vi "initializeArrayElement.vi"(8 "error in (no error)":errorcluster, 9 "arraySize":u16, 10 "arrayRef":refnum<vi>, 11 "Boolean in":refnum<class "Boolean.lvclass">) -> (0 "error out":errorcluster, 3 "Boolean out":refnum<class "Boolean.lvclass">)   [LabVIEW 2016, in "Boolean.lvclass"]
uses:
  Boolean.lvclass
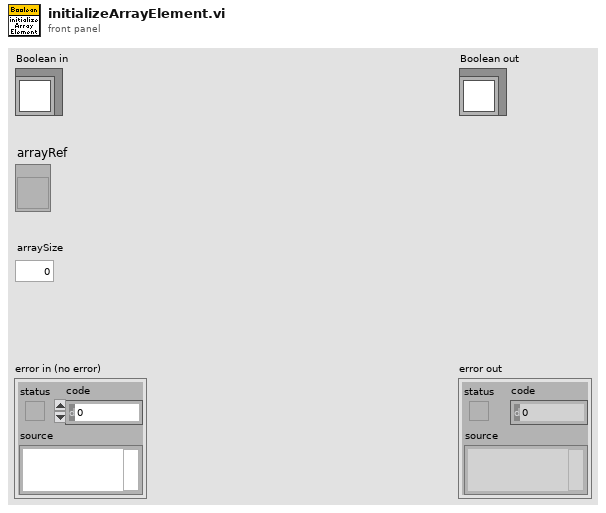
[diagram p1: front panel]
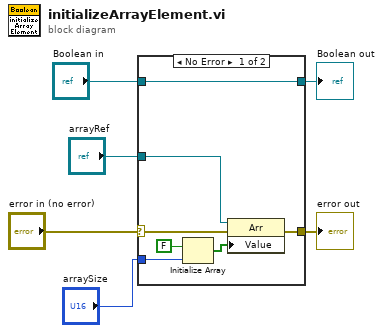
[diagram p0: block diagram]
diagram:
  n1 = case shown="No Error" "error in (no error)" {
    selector: "error in (no error)" -> [w12 w15]
    tunnel: [w11 w15] -> w3
    tunnel: [w10 w14] -> w5
    tunnel: "Boolean in" -> [w10 w14]
    tunnel: "arrayRef" -> [w9 _]
    tunnel: "arraySize" -> [w8 _]
    frame No Error {
      n2 = Initialize Array(FALSE, w8) -> (w13:bool[])
      n3 = property class="Arr"(reference=w9, error in=w12, "Value"=w13) -> (error out=w11:errorcluster)  [unwired: 1 out]
    }
    frame Error {
    }
  }
  "error out" <- w3
  "Boolean out" <- w5
